vi "AlazarCardChannel.vi"(10 "Channel tab":enum32{"C1", "C2", "C3", "C4"}(ring), 11 "Digitizer Settings":T1 {"Trigger Settings"."Trig Slope" items=["Positive", "Negative"]; "Trigger Settings"."Level (mV)" format="%.2f"; "Trigger Settings"."Trig Coupling" items=["DC 1 MOhm", "AC 1 MOhm", "DC 50 Ohm", "AC 50 Ohm"]; "Trigger Settings"."Trig Source" items=["Chan 1", "External"]; "Rel Dig Delay" format="%.2f"; "DigTimeOut" format="%.2f"; "Avg Num" min=1; "Offset delay (us)" format="%.2f"; "Additional dig delay (us)" format="%.2f"; "Digitizer delay (us)" format="%.2f"}) -> (1 "ChansOnOneCard":i32, 2 "Channel":u32, 3 "Card ID":u32)   [LabVIEW 2022 SP3]
uses:
  -DigitizerRoutines/DigitizerSettings.ctl
  -DigitizerRoutines/Digitizer.ctl
  -DigitizerRoutines/DigConfig.ctl
  -DigitizerRoutines/DigitizerID.ctl
  C:/Windows/System32/ADQAPI_dotNet_helper.dll
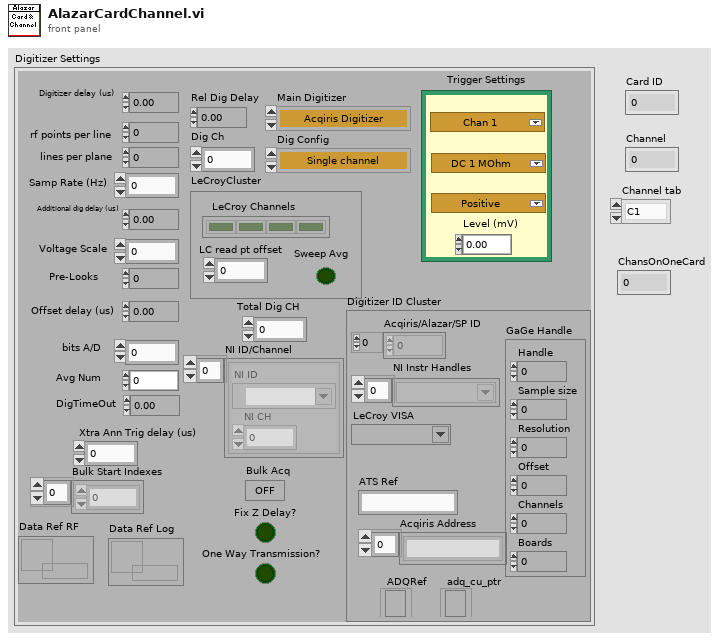
[diagram p1: front panel]
types:
  T1 = typedef "DigitizerSettings.ctl" = cluster{"Digitizer delay (us) ":dbl, "rf points per line":i32, "lines per plane":i32, "Samp Rate (Hz)":dbl, "Additional dig delay (us)":dbl, "Voltage Scale":dbl, "Pre-Looks":i32, "Offset delay (us)":dbl, "bits A/D":i8, "Avg Num":i32, "DigTimeOut":sgl, "Rel Dig Delay":sgl, "Dig Ch":i32, "LeCroyCluster":cluster{"LeCroy Channels":bool[], "LC read pt offset":dbl, "Sweep Avg":bool}, "Main Digitizer":T2, "Dig Config":T3, "Digitizer ID Cluster":T4, "Trigger Settings":cluster{"Trig Source":u16, "Trig Coupling":u16, "Trig Slope":u16, "Level (mV)":dbl}, "Bulk Acq":bool, "Bulk Start Indexes":i32[], "Data Ref RF":refnum<data-value>, "NI ID/Channel":cluster{"NI ID":refnum<k15>, "NI CH":i32}[], "Total Dig CH":i32, "Xtra Ann Trig delay (us)":dbl, "Fix Z Delay?":bool, "One Way Transmission?":bool, "Data Ref Log":refnum<data-value>}
  T2 = typedef "Digitizer.ctl" = enum16{"Acqiris Digitizer", "NI Digitizer", "LeCroy", "GaGe", "AlazarTech", "No Digitizer", "Teledyne"}
  T3 = typedef "DigConfig.ctl" = enum16{"Single channel", "2 Chans w/ 2 Acqiris", "2 Chans w/ 1 Acqiris", "5-CH Pulser New", "5-CH pulser w/ ann array", "5-pass style ann array", "Empty"}
  T4 = typedef "DigitizerID.ctl" = cluster{"Acqiris/Alazar/SP ID":u32[], "NI Instr Handles":refnum<k15>[], "LeCroy VISA":refnum<visa-resource-name>, "GaGe Handle":cluster{"Handle":u32, "Sample size":u32, "Resolution":i32, "Offset":i32, "Channels":u32, "Boards":u32}, "ATS Ref":string, "Acqiris Address":string[], "ADQRef":refnum<k24>, "adq_cu_ptr":refnum<k24>}
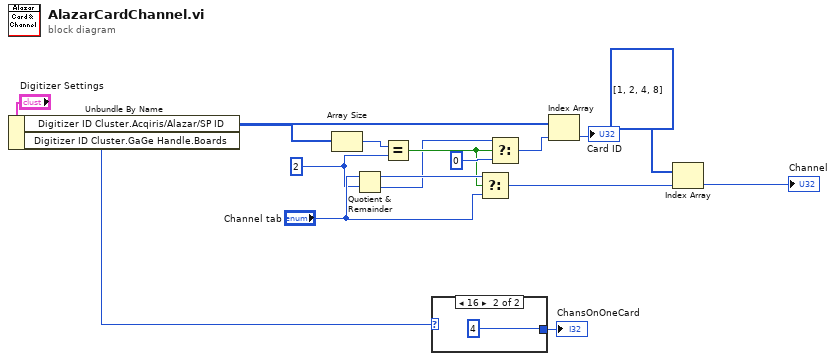
[diagram p0: block diagram]
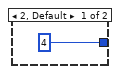
[diagram p2: hidden frame]
diagram:
  w9 = 2
  w5 = u32[] [1, 2, 4, 8] items=["A"=1, "B"=2, "C"=4, "D"=8]
  n1 = Unbundle By Name("Digitizer Settings") -> ("Digitizer ID Cluster.Acqiris/Alazar/SP ID"=w8:u32[], "Digitizer ID Cluster.GaGe Handle.Boards"=w1:u32)
  n2 = Array Size(array=w8) -> (size(s)=w14:i32)
  n3 = Quotient & Remainder(x="Channel tab", y=w9) -> (x-y*floor(x/y)=w12:u32, floor(x/y)=w10:u32)
  n4 = Equal?(x=w14, y=w9) -> (x = y?=w11:bool)
  n5 = case shown="16" w1 {
    tunnel: [4 4] -> w2
    frame 2, Default {
    }
    frame 16 {
    }
  }
  "ChansOnOneCard" <- w2
  n6 = Select(t=w12, s=w11, f="Channel tab") -> (s? t:f=w3:u32)
  n7 = Select(t=w10, s=w11, f=0) -> (s? t:f=w13:u32)
  n8 = Index Array(array=w8, index=w13) -> (element=→"Card ID":u32)
  n9 = Index Array(array=w5, index=w3) -> (element=→"Channel":u32)
